vi "Get Property Description.vi"(0 "SLSC Remote in":refnum<class "SLSC Remote.lvclass">, 5 "property":refnum<k21>, 11 "error in (no error)":errorcluster) -> (4 "SLSC Remote out":refnum<class "SLSC Remote.lvclass">, 6 "property out":refnum<k21>, 10 "Prop.Descr":string, 15 "error out":errorcluster)   [LabVIEW 2016, in "SLSC Interfaces.lvlib" / "SLSC Remote.lvclass"]
uses:
  SLSC Remote.lvclass
  C:/Users/tblair/Documents/Git Projects/SLSC-Interface/Source/SLSC Interface Class/SLSC Interface.lvclass
  <vilib>/National Instruments/JSON Support for LabVIEW/JSON Data Classes/JSON Object/JSON Object.lvclass
  C:/Program Files (x86)/National Instruments/LabVIEW 2016/vi.lib/National Instruments/JSON Support for LabVIEW/JSON Data Classes/JSON Datatype/JSON Datatype.lvclass
  <vilib>/National Instruments/JSON Support for LabVIEW/JSON Data Classes/JSON Object/New JSON Object (Empty).vi
  <vilib>/National Instruments/JSON Support for LabVIEW/JSON Data Classes/JSON Object/Insert Key Value Pair (Single String).vi
  <vilib>/NI/NI JSONRPC Server Framework/Classes/Server/Format Client Request (Auto-Increment).vi
  <vilib>/httpClient/POSTBuffer.vi
  <vilib>/National Instruments/JSON Support for LabVIEW/JSON Data Classes/JSON Datatype/To More Specific Type (Object).vi
  <vilib>/National Instruments/JSON Support for LabVIEW/JSON Data Classes/JSON Object/Get Value (String Value).vi
  <vilib>/NI/NI JSONRPC Server Framework/Classes/Server/JSONRPC Server.lvclass
  <vilib>/httpClient/LabVIEWHTTPClient.lvlib
  <vilib>/National Instruments/JSON Support for LabVIEW/JSON Data Classes/JSON Datatype/JSON Datatype.lvclass
  C:/Program Files (x86)/National Instruments/LabVIEW 2016/vi.lib/National Instruments/JSON Support for LabVIEW/JSON Data Classes/JSON Structured Type/JSON Structured Type.lvclass
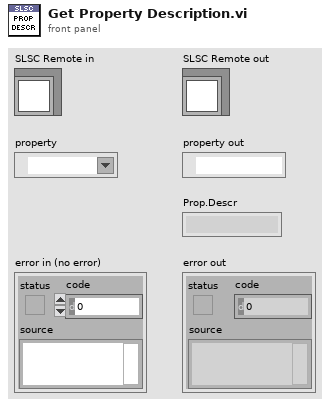
[diagram p1: front panel]
types:
  T1 = typedef "LabVIEWHTTPClient.lvlib/ClientHandle.ctl" = refnum<k1>
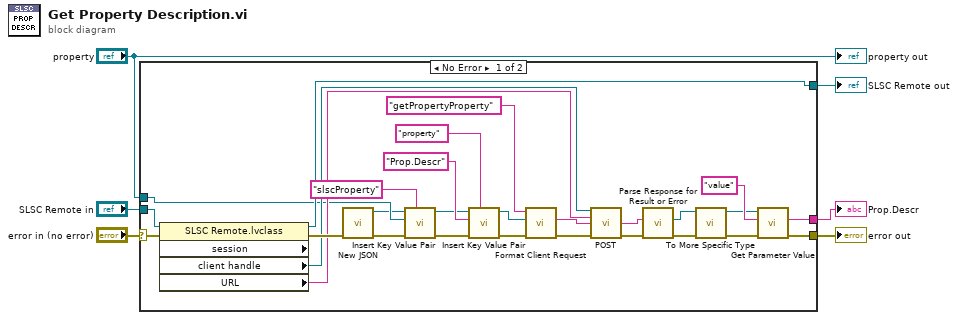
[diagram p0: block diagram]
diagram:
  n1 = case shown="No Error" "error in (no error)" {
    selector: "error in (no error)" -> [w32 w35]
    tunnel: "SLSC Remote in" -> [w34 w36]
    tunnel: [w33 w36] -> w4
    tunnel: [w21 w35] -> w3
    tunnel: [w20 _] -> w1
    tunnel: "property" -> [w12 _]
    frame No Error {
      n2 = property class="SLSC Remote.lvclass" props=["session", "client handle", "URL"](reference=w34, error in=w32) -> (reference out=w33:refnum<class "SLSC Remote.lvclass">, error out=w31:errorcluster, "client handle"=w27:T1, "URL"=w26:string)  [unwired: 1 out]
      n3 = call-poly <vilib>:"New JSON.vi"("error in (no error)"=w31) -> ("error out"=w30:errorcluster, "JSON Object out"=w10:refnum<class "JSON Object.lvclass">)  [unwired: 9 in]
      n4 = call-poly <vilib>:"Insert Key Value Pair.vi"("key"="slscProperty" ("Name"), "error in (no error)"=w30, "value"=w12, "JSON Object in"=w10) -> ("error out"=w16:errorcluster, "JSON Object out"=w11:refnum<class "JSON Object.lvclass">)  [unwired: 5 in, 1 out]
      n5 = call-poly <vilib>:"Insert Key Value Pair.vi"("key"="property" ("Name"), "error in (no error)"=w16, "value"="Prop.Descr" ("String"), "JSON Object in"=w11) -> ("error out"=w18:errorcluster, "JSON Object out"=w19:refnum<class "JSON Object.lvclass">)  [unwired: 5 in, 1 out]
      n6 = call-poly <vilib>:"Format Client Request.vi"("error in (no error)"=w18, "JSON in"=w19, "method"="getPropertyProperty") -> ("error out"=w25:errorcluster, "Request String"=w28:string)  [unwired: 7 in]
      n7 = call-poly <vilib>:"POST.vi"("client handle"=w27, "url"=w26, "buffer"=w28, "error in (no error)"=w25) -> ("body"=w24:string, "error out"=w23:errorcluster)  [unwired: 8 in, 2 out]
      n8 = call <vilib>:"Parse Response for Result or Error.vi"("error in"=w23, "Response String In"=w24) -> ("error out"=w22:errorcluster, "JSON out"=w8:refnum<class "JSON Datatype.lvclass">)  [unwired: 7 in, 1 out]
      n9 = call-poly <vilib>:"To More Specific Type.vi"("error in (no error)"=w22, "JSON Datatype in"=w8) -> ("error out"=w9:errorcluster, "JSON Datatype out"=w7:refnum<class "JSON Object.lvclass">)  [unwired: 8 in]
      n10 = call-poly <vilib>:"Get Parameter Value.vi"("error in (no error)"=w9, "key"="value" ("Parameter Name"), "JSON Object in"=w7) -> ("error out"=w21:errorcluster, "value"=w20:string)  [unwired: 6 in, 1 out]
    }
    frame Error {
    }
  }
  "error out" <- w3
  "SLSC Remote out" <- w4
  "Prop.Descr" <- w1
  "property out" <- "property"
